vi "Calculate BER.vi"(9 "Output Stream":i32[](array[numeric]), 11 "Input Stream":i32[](array[numeric])) -> (3 "BER":dbl)   [LabVIEW 2011]
panel:
  in  "Mapping Parameters":T1={"Modulation Order"=2, "Modulation Type"=0, "Samples per Symbol"=8} {"Modulation Type" items=["PSK", "QAM"]}
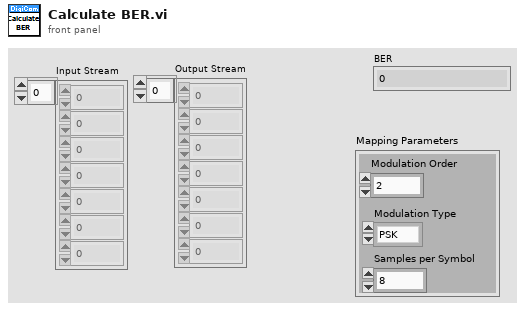
[diagram p1: front panel]
types:
  T1 = cluster{"Modulation Order":i32, "Modulation Type":u16, "Samples per Symbol":i32}
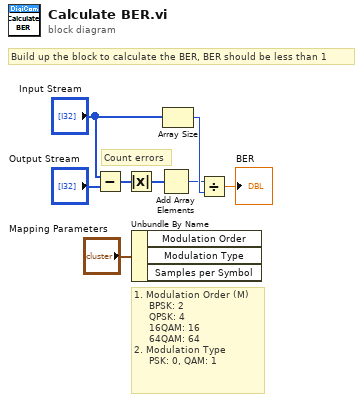
[diagram p0: block diagram]
diagram:
  # "Count errors"
  # "Build up the block to calculate the BER, BER should be less than 1"
  # "1. Modulation Order (M)\n     BPSK: 2\n     QPSK: 4\n     16QAM: 16\n     64QAM: 64\n2. Modulation Type\n     PSK: 0, QAM: 1"
  n1 = Subtract(x="Input Stream", y="Output Stream") -> (x-y=w7:i32[])
  n2 = Absolute Value(x=w7) -> (abs(x)=w3:i32[])
  n3 = Unbundle By Name("Mapping Parameters") -> ()  [unwired: 3 out]
  n4 = Add Array Elements(numeric array=w3) -> (sum=w2:i32)
  n5 = Array Size(array="Input Stream") -> (size(s)=w6:i32)
  n6 = Divide(x=w2, y=w6) -> (x/y=→"BER":dbl)
